vi "READ.vi"(0 "System no.":i32=1 min=1 max=4 step=1, 2 "File name":string, 5 "error in":errorcluster) -> (14 "File contents":string, 19 "error out":errorcluster)   [LabVIEW 2020]
doc: "Reads the contents of the given file.\n\nC-887, F-206, M-8X0: Only for GCS syntax version = GCS 1.0 (Check with CSV?.vi. If CSV?.vi is not supported, syntax version is GCS 1.0). File name can be any file stored on the controller with file extension .dat, .txt or .mac. For files outside the HEXAPOD directory the full path must be given."
panel:
  # "Reads the contents of the given file."
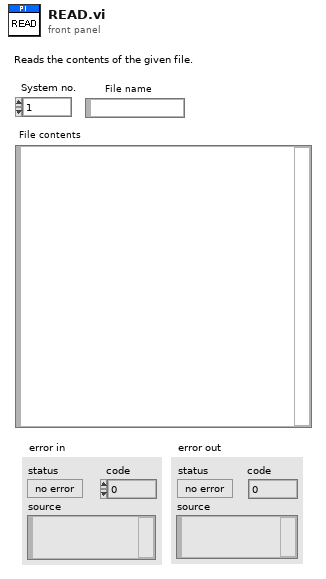
[diagram p1: front panel]
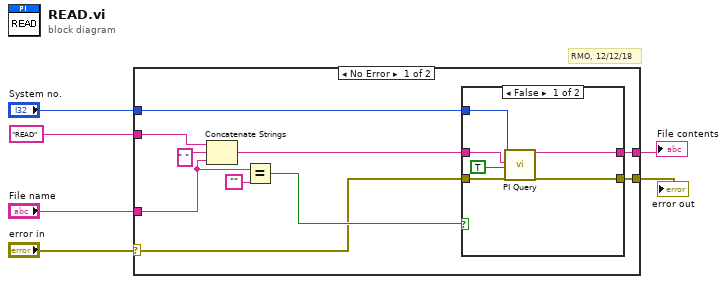
[diagram p0: block diagram]
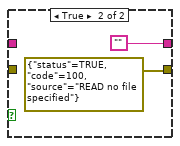
[diagram p2: hidden frame]
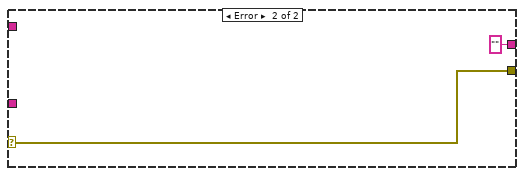
[diagram p3: hidden frame]
diagram:
  # "RMO, 12/12/18"
  n1 = case shown="No Error" "error in" {
    selector: "error in" -> [w7 w25]
    tunnel: [w16 "" ("String read")] -> w6
    tunnel: [w15 w25] -> w5
    tunnel: "System no." -> [w14 _]
    tunnel: "READ" ("String to Send") -> [w13 _]
    tunnel: "File name" -> [w12 _]
    frame No Error {
      n2 = Concatenate Strings(w13, " ", w12) -> (w11:string)
      n3 = Equal?(x=w12, y="") -> (x = y?=w10:bool)
      n4 = case shown="False" w10 {
        tunnel: [w17 ""] -> w16
        tunnel: [w18 errorcluster {"status"=TRUE, "code"=100, "source"="READ no file specified"} ("error out")] -> w15
        tunnel: w14 -> [w20 _]
        tunnel: w7 -> [w21 _]
        tunnel: w11 -> [w19 _]
        frame False {
          n5 = call "PI Query.vi"("System no."=w20, "String to send"=w19, "Attach termination char.?"=TRUE ("Attach Linefeed?"), "error in"=w21) -> ("String read"=w17:string, "error out"=w18:errorcluster)  [unwired: 3 in, 11 out]
        }
        frame True {
        }
      }
    }
    frame Error {
    }
  }
  "File contents" <- w6
  "error out" <- w5
